vi "Kill.vi"(7 "timeout [ms]":i32, 8 "error in":errorcluster, 11 "pipe in":T1) -> (0 "error out":errorcluster, 3 "pipe out":T1)   [LabVIEW 2013]
doc: "Calls lv_proc.dll to kill process. This VI is recommended to use only if there is no other way how to force process exit."
uses:
  Pipe Handle.ctl
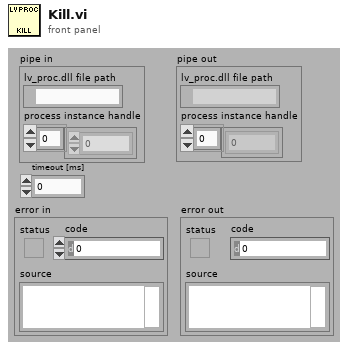
[diagram p1: front panel]
types:
  T1 = typedef "Pipe Handle.ctl" = cluster{"lv_proc.dll file path":path, "process instance handle":u32[]}
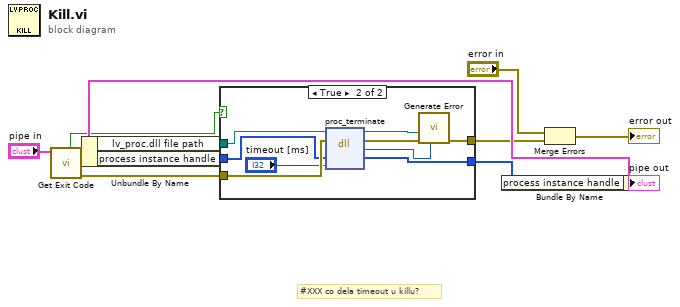
[diagram p0: block diagram]
diagram:
  # "#XXX co dela timeout u killu?"
  n1 = call "Get Exit Code.vi"("pipe in"="pipe in") -> ("error out"=w4:errorcluster, "pipe out"=w7:T1, "running?"=w6:bool)  [unwired: 6 in, 2 out]
  n2 = Unbundle By Name(w7) -> ("lv_proc.dll file path"=w11:path, "process instance handle"=w5:u32[])
  n3 = case shown="True" w6 {
    tunnel: [w12 w15] -> w3
    tunnel: w4 -> [w12 w22]
    tunnel: w5 -> [w13 w21]
    tunnel: [w13 w14] -> w9
    tunnel: w11 -> [_ w19]
    frame False {
    }
    frame True {
      n4 = dll-call lib="lv_proc.dll" fn="proc_terminate"(path in=w19, error in=w22, "proc"=w21, "timeout [ms]"="timeout [ms]") -> (path out=w16:path, error out=w17:errorcluster, "error"=w18:i32, "proc"=w14:u32[])  [unwired: 2 in]
      n5 = call "Generate Error.vi"("error code in"=w18, "error in"=w17, "lv_proc.dll path in"=w16) -> ("error out"=w15:errorcluster)  [unwired: 6 in, 1 out]
    }
  }
  n6 = Bundle By Name(cluster=w7, "process instance handle"=w9) -> (→"pipe out":T1)
  n7 = Merge Errors("error in", w3) -> (→"error out":errorcluster)
